vi "Close RS485.vi"(8 "error in (no error)":errorcluster, 10 "Internal?":bool, 11 "Huber Unistat 410 Settings":T1 {"Address" min=0 max=99 format="%02.0f"}) -> (0 "error out":errorcluster, 3 "Huber Unistat 410 Settings":T1 {"Address" min=0 max=99 format="%02.0f"})   [LabVIEW 2021, in "Huber Unistat 410 TCU.lvlib"]
uses:
  Huber Unistat 410 TCU.lvlib
  Huber Unistat 410 RS485 Settings.ctl
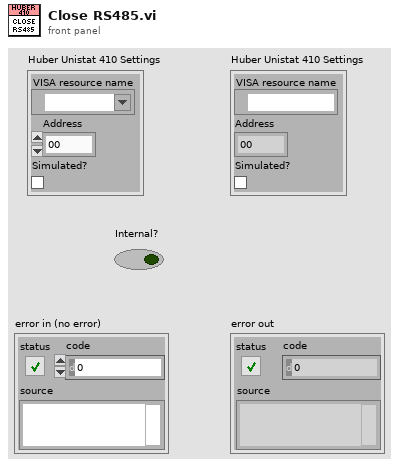
[diagram p1: front panel]
types:
  T1 = typedef "Huber Unistat 410 TCU.lvlib/Huber Unistat 410 RS485 Settings.ctl" = cluster{"VISA resource name":refnum<visa-resource-name>, "Address":i8, "Simulated?":bool}
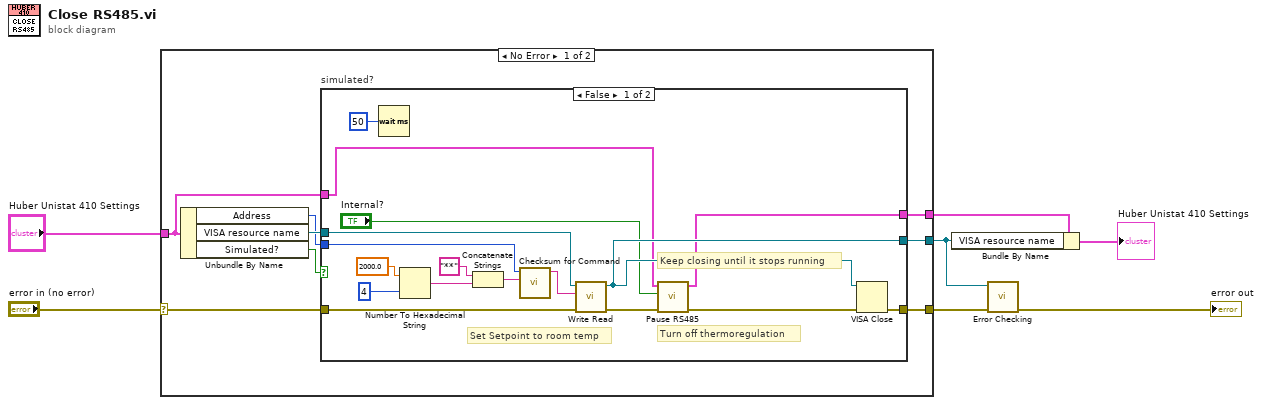
[diagram p0: block diagram]
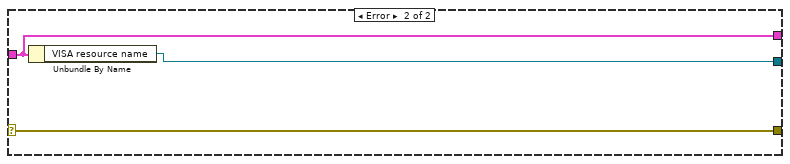
[diagram p3: hidden frame]
diagram:
  n1 = case shown="No Error" "error in (no error)" {
    selector: "error in (no error)" -> [w13 w38]
    tunnel: [w14 w38] -> w6
    tunnel: "Huber Unistat 410 Settings" -> [w10 w36]
    tunnel: [w11 w37] -> w4
    tunnel: [w9 w36] -> w3
    frame No Error {
      n2 = Unbundle By Name(w10) -> ("Address"=w8:i8, "VISA resource name"=w12:refnum<visa-resource-name>, "Simulated?"=w15:bool)
      n3 = case "simulated?" shown="False" w15 {
        tunnel: [w30 w35] -> w14
        tunnel: w12 -> [w29 w34]
        tunnel: w13 -> [w32 w35]
        tunnel: [w28 w34] -> w11
        tunnel: w10 -> [w27 w33]
        tunnel: [w16 w33] -> w9
        tunnel: w8 -> [w26 _]
        frame False {
          # "Turn off thermoregulation"
          # "Set Setpoint to room temp"
          # "Keep closing until it stops running"
          n4 = Wait (ms)(milliseconds to wait=u32 50) -> ()  [unwired: 1 out]
          n5 = Number To Hexadecimal String(1:i16 4 ("width (-)"), 2:2000.0 ("x")) -> (0:w23:string)
          n6 = Concatenate Strings("**" ("string"), w23) -> (w20:string)
          n7 = call "Checksum for Command.vi"("Message"=w20, "Address"=w26) -> ("Formated Message"=w19:string)  [unwired: 9 in]
          n8 = call "Write Read.vi"("error in (no error)"=w32, "write string"=w19, "VISA Refnum in"=w29) -> ("error out"=w17:errorcluster, "VISA Refnum out"=w28:refnum<visa-resource-name>)  [unwired: 6 in, 1 out]
          n9 = call "Pause RS485.vi"("error in (no error)"=w17, "Internal?"="Internal?", "Huber Unistat 410 Settings"=w27) -> ("error out"=w31:errorcluster, "Huber Unistat 410 Settings"=w16:T1)  [unwired: 7 in]
          n10 = VISA Close(VISA resource name=w28, error in (no error)=w31) -> (error out=w30:errorcluster)
        }
        frame True {
        }
      }
    }
    frame Error {
      n11 = Unbundle By Name(w36) -> ("VISA resource name"=w37:refnum<visa-resource-name>)
    }
  }
  n12 = Bundle By Name(cluster=w3, "VISA resource name"=w4) -> (→"Huber Unistat 410 Settings":T1)
  n13 = call "Error Checking.vi"("error in (no error)"=w6, "VISA resource name"=w4) -> ("error out"=→"error out":errorcluster)  [unwired: 7 in, 2 out]
